vi "DisableUIButtons.vi"(10 "reference":refnum<vi>) -> ()   [LabVIEW 2023, in "InterferometrUI.lvlib" / "InterferometerUI.lvclass"]
uses:
  InterferometerUI.lvclass
  InterferometerUI.lvclass/InterferometerUI.ctl
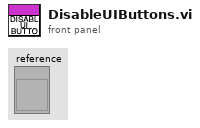
[diagram p1: front panel]
types:
  T1 = enum8{"Enabled", "Disabled", "Disabled and Grayed Out"}
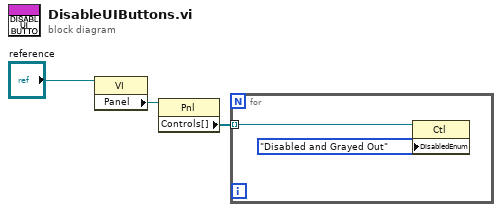
[diagram p0: block diagram]
diagram:
  n1 = property on="Property Node" class="VI"(reference="reference") -> ("Panel"=w3:refnum<vi>)  [unwired: 1 in, 2 out]
  n2 = property on="Property Node" class="Pnl"(reference=w3) -> ("Controls[]"=w2:refnum<vi>[])  [unwired: 1 in, 2 out]
  n3 = for {
    tunnel: w2 -> [w5] mode=indexing
    n4 = property on="Property Node" class="Ctl"(reference=w5, "DisabledEnum"=T1."Disabled and Grayed Out" ("Disabled")) -> ()  [unwired: 1 in, 2 out]
  }
